vi "Read body.vi"(11 "httpResponse in":refnum<class "httpResponse.lvclass">) -> (2 "body":string, 3 "httpResponse out":refnum<class "httpResponse.lvclass">)   [LabVIEW 2020, in "httpClient.lvlib" / "httpResponse.lvclass"]
uses:
  httpResponse.lvclass
  httpResponse.lvclass/httpResponse.ctl
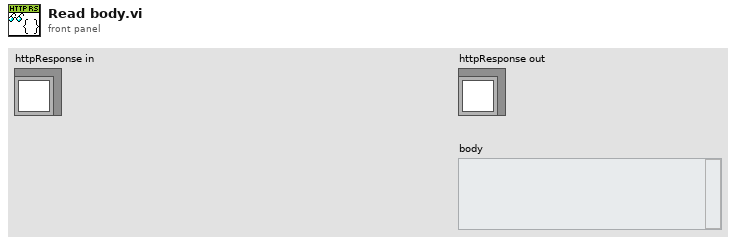
[diagram p1: front panel]
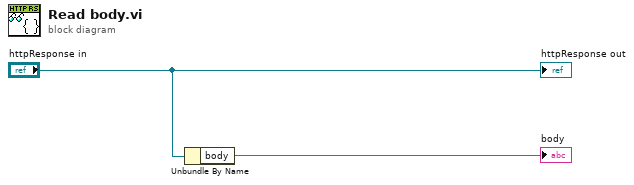
[diagram p0: block diagram]
diagram:
  n1 = Unbundle By Name("httpResponse in") -> ("body"=→"body":string)
  "httpResponse out" <- "httpResponse in"
